vi "Read spectId.vi"(8 "error in (no error)":errorcluster, 11 "StopImageCapture in":refnum<class "StopImageCapture.lvclass">) -> (0 "error out":errorcluster, 2 "spectId":u16, 3 "StopImageCapture out":refnum<class "StopImageCapture.lvclass">)   [LabVIEW 2016, in "Commands.lvlib" / "StopImageCapture.lvclass"]
uses:
  StopImageCapture.lvclass
  StopImageCapture.lvclass/StopImageCapture.ctl
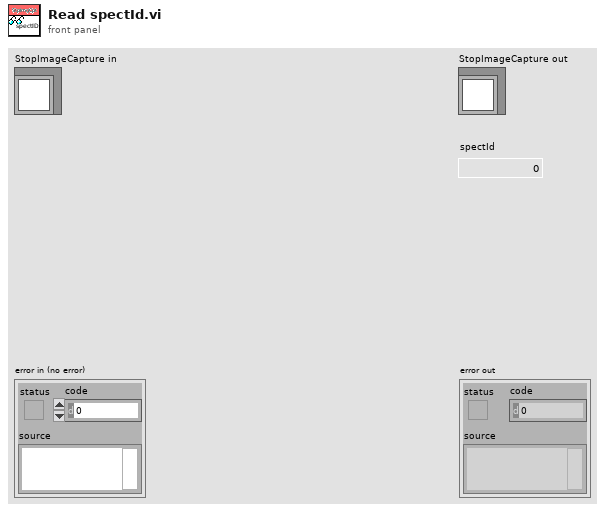
[diagram p1: front panel]
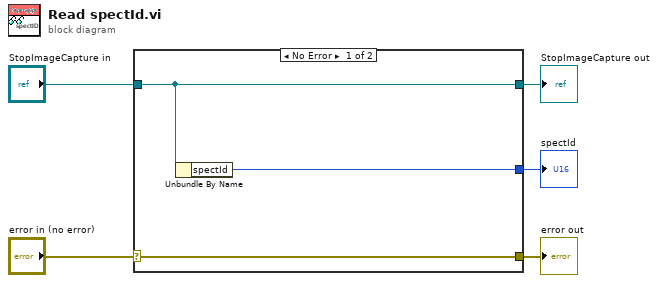
[diagram p0: block diagram]
diagram:
  n1 = case shown="No Error" "error in (no error)" {
    selector: "error in (no error)" -> [w8 w9]
    tunnel: [w8 w9] -> w4
    tunnel: [w7 w10] -> w2
    tunnel: "StopImageCapture in" -> [w7 w10]
    tunnel: [w6 _] -> w1
    frame No Error {
      n2 = Unbundle By Name(w7) -> ("spectId"=w6:u16)
    }
    frame Error {
    }
  }
  "error out" <- w4
  "StopImageCapture out" <- w2
  "spectId" <- w1
